vi "Destroy.vi"(0 "reference in":refnum<class "CompositeIterator.lvclass">, 5 "error in (no error)":errorcluster) -> (14 "reference out":refnum<class "CompositeIterator.lvclass">, 19 "error out":errorcluster)   [LabVIEW 2015, in "CompositeIterator.lvclass"]
uses:
  CompositeIterator.lvclass
  Interface/Iterator.lvclass
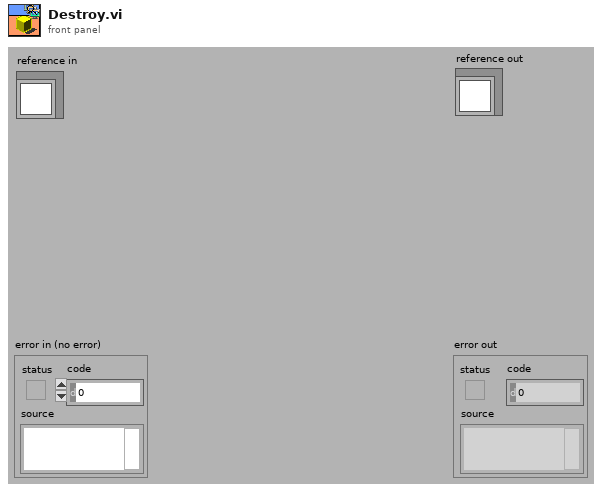
[diagram p1: front panel]
types:
  T1 = typedef "CompositeIterator.lvclass/ObjectAttributes.ctl" = cluster{"Stack":refnum<queue>}
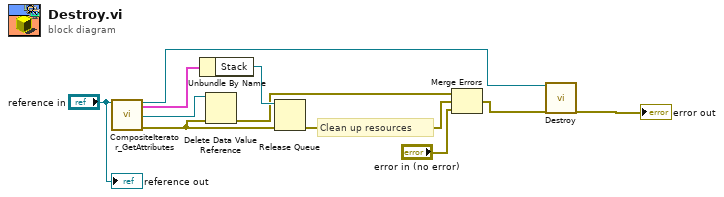
[diagram p0: block diagram]
diagram:
  # "Clean up resources"
  n1 = call "CompositeIterator_GetAttributes.vi"("reference in"="reference in") -> ("reference out"=w2:refnum<class "CompositeIterator.lvclass">, "Data"=w7:T1, "DataRef"=w6:refnum<data-value>, "error out"=w5:errorcluster)  [unwired: 15 in]
  n2 = Unbundle By Name(w7) -> ("Stack"=w10:refnum<queue>)
  n3 = Delete Data Value Reference(data value reference=w6, error in=w5) -> (error out=w4:errorcluster)  [unwired: 1 out]
  n4 = Release Queue(queue=w10, error in (no error)=w5) -> (error out=w9:errorcluster)  [unwired: 1 in, 2 out]
  n5 = Merge Errors(w4, w9, "error in (no error)") -> (w3:errorcluster)
  n6 = call-parent "Destroy.vi"("reference in"=w2, "error in (no error)"=w3) -> ("error out"=→"error out":errorcluster)  [unwired: 16 in, 1 out]
  "reference out" <- "reference in"
